vi "Skeletonized Watershed.vi"(9 "Image Name":string="untitled", 10 "Connectivity 4/8 (4)":bool, 11 "Grayscale Image":T2) -> (0 "Particle Reports (Pixels)":T1(array[cluster]) {"Orientation" format="%.2f"; "Dimensions"."Height" format="%.2f"; "Dimensions"."Width" format="%.2f"; "Center of Mass"."Y" format="%.2f"; "Center of Mass"."X" format="%.2f"; "Bounding Rect"."Bottom" format="%.2f"; "Bounding Rect"."Right" format="%.2f"; "Bounding Rect"."Top" format="%.2f"; "Bounding Rect"."Left" format="%.2f"; "Number of Holes" format="%.2f"; "Area" format="%.2f"}, 1 "Number of Zones":i32, 3 "Image Out":T2)   [LabVIEW 2018]
uses:
  <vilib>/vision/Image Controls.llb/IMAQ Image.ctl
  <vilib>/vision/NI_Vision_Development_Module.lvlib
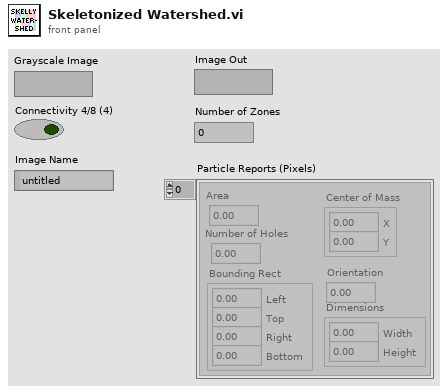
[diagram p1: front panel]
types:
  T1 = cluster{"Area":dbl, "Number of Holes":dbl, "Bounding Rect":cluster{"Left":dbl, "Top":dbl, "Right":dbl, "Bottom":dbl}, "Center of Mass":cluster{"X":dbl, "Y":dbl}, "Orientation":dbl, "Dimensions":cluster{"Width":dbl, "Height":dbl}}[]
  T2 = typedef "IMAQ Image.ctl" = refnum<image>
  T3 = typedef "Image Type" = u32
  T4 = enum32{"Differentiation", "Gradient", "Prewitt", "Roberts", "Sigma", "Sobel"}
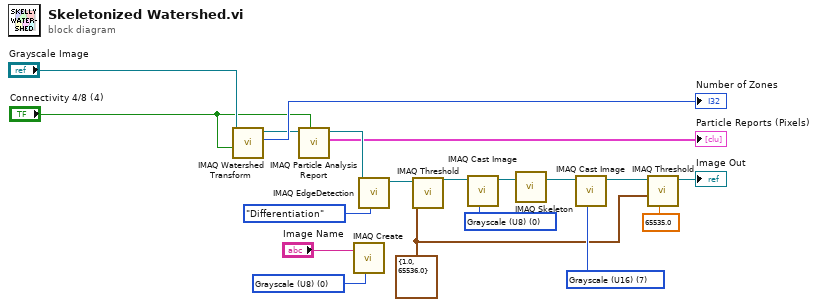
[diagram p0: block diagram]
diagram:
  w6 = cluster{"Lower value":sgl, "Upper value":sgl} {"Lower value"=1.0, "Upper value"=65536.0} ("Range")
  w9 = T3 7 items=["Grayscale (U8)", "Grayscale (I16)", "Grayscale (SGL)", "Complex (CSG)", "RGB (U32)", "HSL (U32)", "RGB (U64)", "Grayscale (U16)"] ("Image Type")
  w11 = T3 0 items=["Grayscale (U8)", "Grayscale (I16)", "Grayscale (SGL)", "Complex (CSG)", "RGB (U32)", "HSL (U32)", "RGB (U64)", "Grayscale (U16)"] ("Image Type")
  w14 = T3 0 items=["Grayscale (U8)", "Grayscale (I16)", "Grayscale (SGL)", "Complex (CSG)", "RGB (U32)", "HSL (U32)", "RGB (U64)", "Grayscale (U16)"] ("Image Type")
  n1 = call "IMAQ Watershed Transform"("Connectivity 4/8 (8)"="Connectivity 4/8 (4)", "Image Src"="Grayscale Image") -> ("Number Of Zones"=→"Number of Zones":i32, "Image Dst Out"=w4:T2)  [unwired: 7 in, 1 out]
  n2 = call "IMAQ Particle Analysis Report"("Connectivity 4/8 (8)"="Connectivity 4/8 (4)", "Image"=w4) -> ("Particle Reports (Pixels)"=→"Particle Reports (Pixels)":T1, "Image Out (duplicate)"=w3:T2)  [unwired: 4 in, 4 out]
  n3 = call "IMAQ Create"("Image Name"="Image Name", "Image Type"=w14) -> ()  [unwired: 3 in, 2 out]
  n4 = call "IMAQ EdgeDetection"("Method"=T4."Differentiation", "Image Src"=w3) -> ("Image Dst Out"=w18:T2)  [unwired: 8 in, 1 out]
  n5 = call "IMAQ Threshold"("Range"=w6, "Image Src"=w18) -> ("Image Dst Out"=w13:T2)  [unwired: 8 in, 1 out]
  n6 = call "IMAQ Cast Image"("Image Type"=w11, "Image Src"=w13) -> ("Image Dst Out"=w12:T2)  [unwired: 8 in, 1 out]
  n7 = call "IMAQ Skeleton"("Image Src"=w12) -> ("Image Dst Out"=w10:T2)  [unwired: 5 in, 1 out]
  n8 = call "IMAQ Cast Image"("Image Type"=w9, "Image Src"=w10) -> ("Image Dst Out"=w8:T2)  [unwired: 8 in, 1 out]
  n9 = call "IMAQ Threshold"("Replace Value"=sgl 65535.0, "Range"=w6, "Image Src"=w8) -> ("Image Dst Out"=→"Image Out":T2)  [unwired: 7 in, 1 out]
